vi "PruebaAutoR.vi"() -> ()   [LabVIEW 2014, in "MSX-E3701_dll.lvlib"]
uses:
  MSX-E3701_dll.lvlib
  Typedef/Config Data.ctl
  Typedef/Connection Data.ctl
  E:/Repositorio Magnis/INF002/v0/Modules/HAL/Drivers/Sync/ADDI-DATA MSX-E3701/API/MX370x.dll
  MX370x.dll
  E:/Repositorio Magnis/INF002/v0/Modules/HAL/Drivers/Sync/ADDI-DATA MSX-E3701/API/MXCommon.dll
  MXCommon.dll
  Typedef/Adquisition Data.ctl
panel:
  out "error out":errorcluster
  in  "error in (no error)":errorcluster
  in  "Transductores":bool[][](array[boolean])
  out "Casteado":sgl[](array[numeric])
  out "Adquisition Data":T1
  in  "stop":bool
  in  "Connection Data In":T2
  in  "Config Data":T3
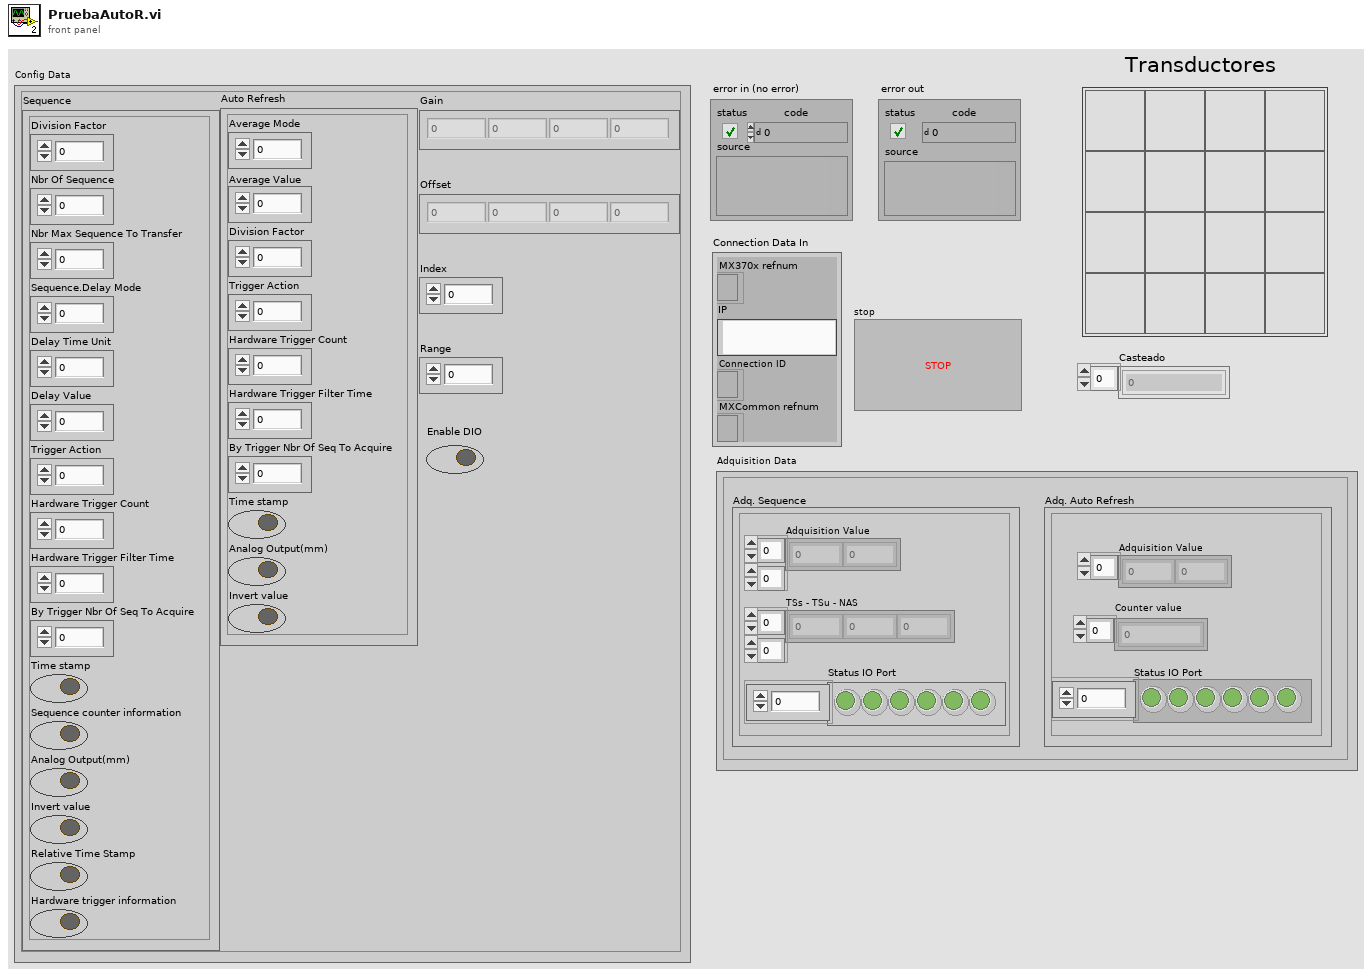
[diagram p1: front panel]
types:
  T1 = typedef "MSX-E3701_dll.lvlib/Adquisition Data.ctl" = cluster{"Adq. Sequence":cluster{"TSs - TSu - NAS":u64[][], "Adquisition Value":u32[][], "Status IO Port":bool[]}, "Adq. Auto Refresh":cluster{"Adquisition Value":u64[], "Status IO Port":bool[], "Counter value":u64[]}}
  T2 = typedef "MSX-E3701_dll.lvlib/Connection Data.ctl" = cluster{"MX370x refnum":refnum<k24>, "IP":string, "Connection ID ":refnum<k5>, "MXCommon refnum":refnum<k24>}
  T3 = typedef "MSX-E3701_dll.lvlib/Config Data.ctl" = cluster{"Auto Refresh":cluster{"Average Mode":u64, "Average Value":u64, "Division Factor":u64, "Trigger Action":u64, "Hardware Trigger Count":u64, "Hardware Trigger Filter Time":u64, "By Trigger Nbr Of Seq To Acquire":u64, "Time stamp":bool, "Analog Output(mm)":bool, "Invert value":bool}, "Gain":sgl[], "Offset":sgl[], "Index":u64, "Range":sgl, "Sequence":cluster{"Division Factor":u64, "Nbr Of Sequence":u64, "Nbr Max Sequence To Transfer":u64, "Sequence.Delay Mode":u64, "Delay Time Unit":u64, "Delay Value":u64, "Trigger Action":u64, "Hardware Trigger Count":u64, "Hardware Trigger Filter Time":u64, "By Trigger Nbr Of Seq To Acquire":u64, "Time stamp":bool, "Sequence counter information":bool, "Analog Output(mm)":bool, "Invert value":bool, "Relative Time Stamp":bool, "Hardware trigger information":bool}, "Enable DIO":bool}
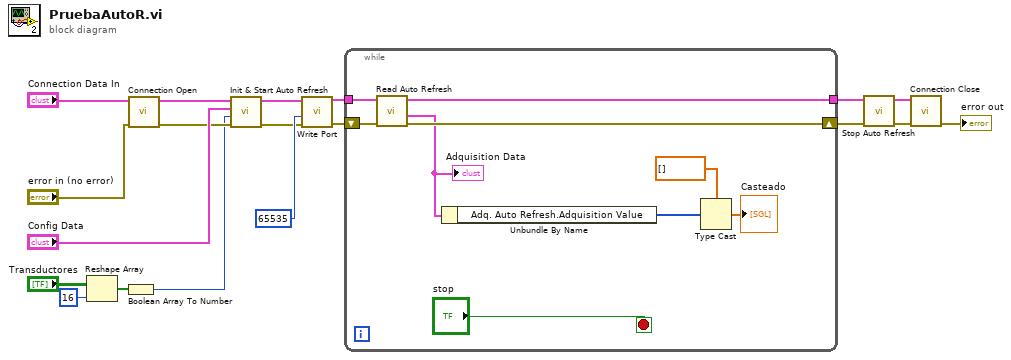
[diagram p0: block diagram]
diagram:
  n1 = Reshape Array("Transductores", 16 ("dimension size")) -> (w6:bool[])
  n2 = Boolean Array To Number(Boolean array=w6) -> (number=w3:u64)
  n3 = call "Connection Open.vi"("Error In"="error in (no error)", "Connection Data In"="Connection Data In") -> ("Error Out"=w16:errorcluster, "Connection Data Out"=w18:T2)  [unwired: 8 in]
  n4 = call "Init & Start Auto Refresh.vi"("error in (no error)"=w16, "Channel Mask"=w3, "Config Data"="Config Data", "Connection Data In"=w18) -> ("error out"=w9:errorcluster, "Connection Data Out"=w8:T2)  [unwired: 6 in]
  n5 = call "Write Port.vi"("error in (no error)"=w9, "Port Mask"=u64 65535, "Connection Data In"=w8) -> ("error out"=w10:errorcluster, "Connection Data Out"=w7:T2)  [unwired: 7 in]
  n6 = while {
    shift-right: [w27] -> w14
    shift-left: w10 -> [w24]
    tunnel: w7 -> [w25]
    tunnel: [w26] -> w15
    stop <- "stop" stop-if-true
    n7 = call "Read Auto Refresh.vi"("error in (no error)"=w24, "Connection Data In"=w25) -> ("error out"=w27:errorcluster, "Adquisition Data Out"=w23:T1, "Connection Data Out"=w26:T2)  [unwired: 7 in]
    "Adquisition Data" <- w23
    n8 = Unbundle By Name(w23) -> ("Adq. Auto Refresh.Adquisition Value"=w22:u64[])
    n9 = Type Cast(type=sgl[] [], x=w22) -> (*(type *) &x=→"Casteado":sgl[])
  }
  n10 = call "Stop Auto Refresh.vi"("error in (no error)"=w14, "Connection Data In"=w15) -> ("error out"=w12:errorcluster, "Connection Data Out"=w13:T2)  [unwired: 8 in]
  n11 = call "Connection Close.vi"("error in (no error)"=w12, "Connection Data In"=w13) -> ("error out"=→"error out":errorcluster)  [unwired: 8 in, 1 out]
